vi "Мультиплексор(3 одноразрядных операнда).vi"(1 "c":cluster{"c0":bool, "c1":bool}, 2 "x2":bool, 3 "x1":bool, 4 "x0":bool) -> (0 "r":bool)   [LabVIEW 2012]
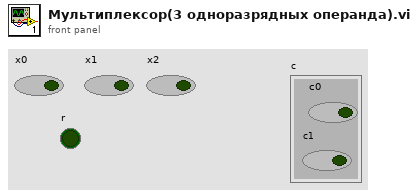
[diagram p1: front panel]
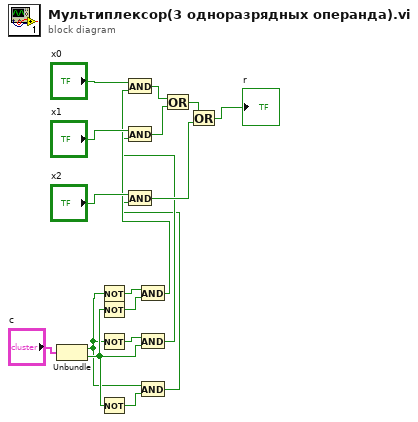
[diagram p0: block diagram]
diagram:
  n1 = Unbundle("c") -> ("c0"=w1:bool, "c1"=w2:bool)
  n2 = Not(x=w1) -> (.not. x?=w9:bool)
  n3 = Not(x=w2) -> (.not. x?=w8:bool)
  n4 = Not(x=w1) -> (.not. x?=w7:bool)
  n5 = Not(x=w2) -> (.not. x?=w6:bool)
  n6 = And(x=w9, y=w8) -> (x .and. y?=w5:bool)
  n7 = And(x="x0", y=w5) -> (x .and. y?=w16:bool)
  n8 = And(x=w7, y=w2) -> (x .and. y?=w4:bool)
  n9 = And(x="x1", y=w4) -> (x .and. y?=w15:bool)
  n10 = And(x=w1, y=w6) -> (x .and. y?=w3:bool)
  n11 = And(x="x2", y=w3) -> (x .and. y?=w12:bool)
  n12 = Or(x=w16, y=w15) -> (x .or. y?=w13:bool)
  n13 = Or(x=w13, y=w12) -> (x .or. y?=→"r":bool)
